vi "CameraSerialController_Experiment5555.vi"() -> (4 "图像时间戳":u32=16532020 format="%_32g")   [LabVIEW 2015]
uses:
  <vilib>/Instr/_visa.llb/VISA Configure Serial Port (Instr).vi
  MVCAMSDK.dll
  <vilib>/Analysis/NI_AALBase.lvlib
panel:
  out "光强图 4":dbl[](graph)
  out "variance 4":dbl caption="方差" format="%0.2f"
  out "光强图 3":dbl[](graph)
  out "variance 3":dbl caption="方差" format="%0.2f"
  out "连接的字符串":string
  out "转动信号曲线":cluster{"Locations":dbl[], "Amplitudes":dbl[]}[](graph)=[{"Locations"=array[750 elements], "Amplitudes"=array[749 elements]}, {"Locations"=[104.38621227921368, 258.3247060234782, 410.71523318402836, 562.6858730022967, 712.7065754646931], "Amplitudes"=[11153.698204083417, 10559.387052180104, 10974.865031894917, 10500.852817232146, 11059.763900010517]}, {"Locations"=[26.787398227992274, 182.39455189327623, 333.5517219531509, 488.1851999460032, 636.5270621135614], "Amplitudes"=[3284.809720018355, 2039.4564261182056, 3638.2587716464914, 3082.2730888167225, 4217.856016996603]}]
  in  "平移回退":T1=TRUE
  in  "转动回退":T1=TRUE
  in  "转动计数":u16
  in  "转动一次脉冲数":u16=20
  in  "转动前进":T1=TRUE
  in  "平移一次脉冲数":u16=20
  in  "平移计数":u16
  out "variance 2":dbl caption="方差" format="%0.2f"
  in  "flow control (0:none)":u16(ring) caption="流控制（0:无）" items=["无", "XON/XOFF", "RTS/CTS", "XON/XOFF & RTS/CTS", "DTR/DSR", "XON/XOFF & DTR/DSR"]
  in  "stop bits (10: 1 bit)":u16=10 caption="停止位（10: 1位）"
  in  "奇偶 (0:none)":enum16{"None", "Odd", "Even", "Mark", "Space"}(ring) caption="奇偶（0:无）"
  in  "数据比特(默认8)":u16(ring)=8 items=["5"=5, "6"=6, "7"=7, "8"=8]
  in  "波特率(默认9600)":u32=9600
  in  "端口":refnum<visa-resource-name>="COM1"
  in  "平移前进":T1=TRUE
  out "泰伯距离数值":dbl[](array[numeric])=[15.393849374426454, 15.239052716055017, 15.197063981826837, 15.002070246239633]
  out "Locations":dbl[](array[numeric])=[10.438621227921368, 25.832470602347822, 41.07152331840284, 56.268587300229676, 71.27065754646931] caption="上面图像曲线波峰位置"
  out "平移信号曲线":cluster{"Locations":dbl[], "Amplitudes":dbl[]}[](graph)=[{"Locations"=array[750 elements], "Amplitudes"=array[749 elements]}, {"Locations"=[104.38621227921368, 258.3247060234782, 410.71523318402836, 562.6858730022967, 712.7065754646931], "Amplitudes"=[11153.698204083417, 10559.387052180104, 10974.865031894917, 10500.852817232146, 11059.763900010517]}, {"Locations"=[26.787398227992274, 182.39455189327623, 333.5517219531509, 488.1851999460032, 636.5270621135614], "Amplitudes"=[3284.809720018355, 2039.4564261182056, 3638.2587716464914, 3082.2730888167225, 4217.856016996603]}]
  out "光强图 2":dbl[](graph)
  out "variance":dbl caption="方差" format="%0.2f"
  out "相机图像":T2(plugin-control)
  out "光强图":dbl[](graph)
  out "帧速":u32
  out "帧间耗时\n单位：（0.1ms）":u32
  in  "相机枚举":T3(ring)
  in  "自动曝光模式":bool=TRUE caption="软触发"
  in  "手动曝光模式":bool caption="软触发"
  in  "曝光时间，单位微秒":dbl=11000.0 format="%#_6f"
  in  "硬触发模式":bool caption="软触发"
  in  "软触发模式":bool caption="软触发"
  in  "连续模式":bool caption="软触发"
  in  "软触发一帧":bool caption="软触发"
  in  "读取自定义数据":bool
  out "从相机中读出的字符串(32字节)":string
  in  "写入自定义数据":bool
  in  "要写入相机的字符串(32字节)":string
  in  "拍照":bool
  in  "相机参数":bool=TRUE
  in  "Stop":bool
  in  "激活预览":bool=TRUE
  out "Image":T2(plugin-control)
  # "相机原生分辨率设置"
  # "写入自定义数据"
  # "触发设置"
  # "曝光设置"
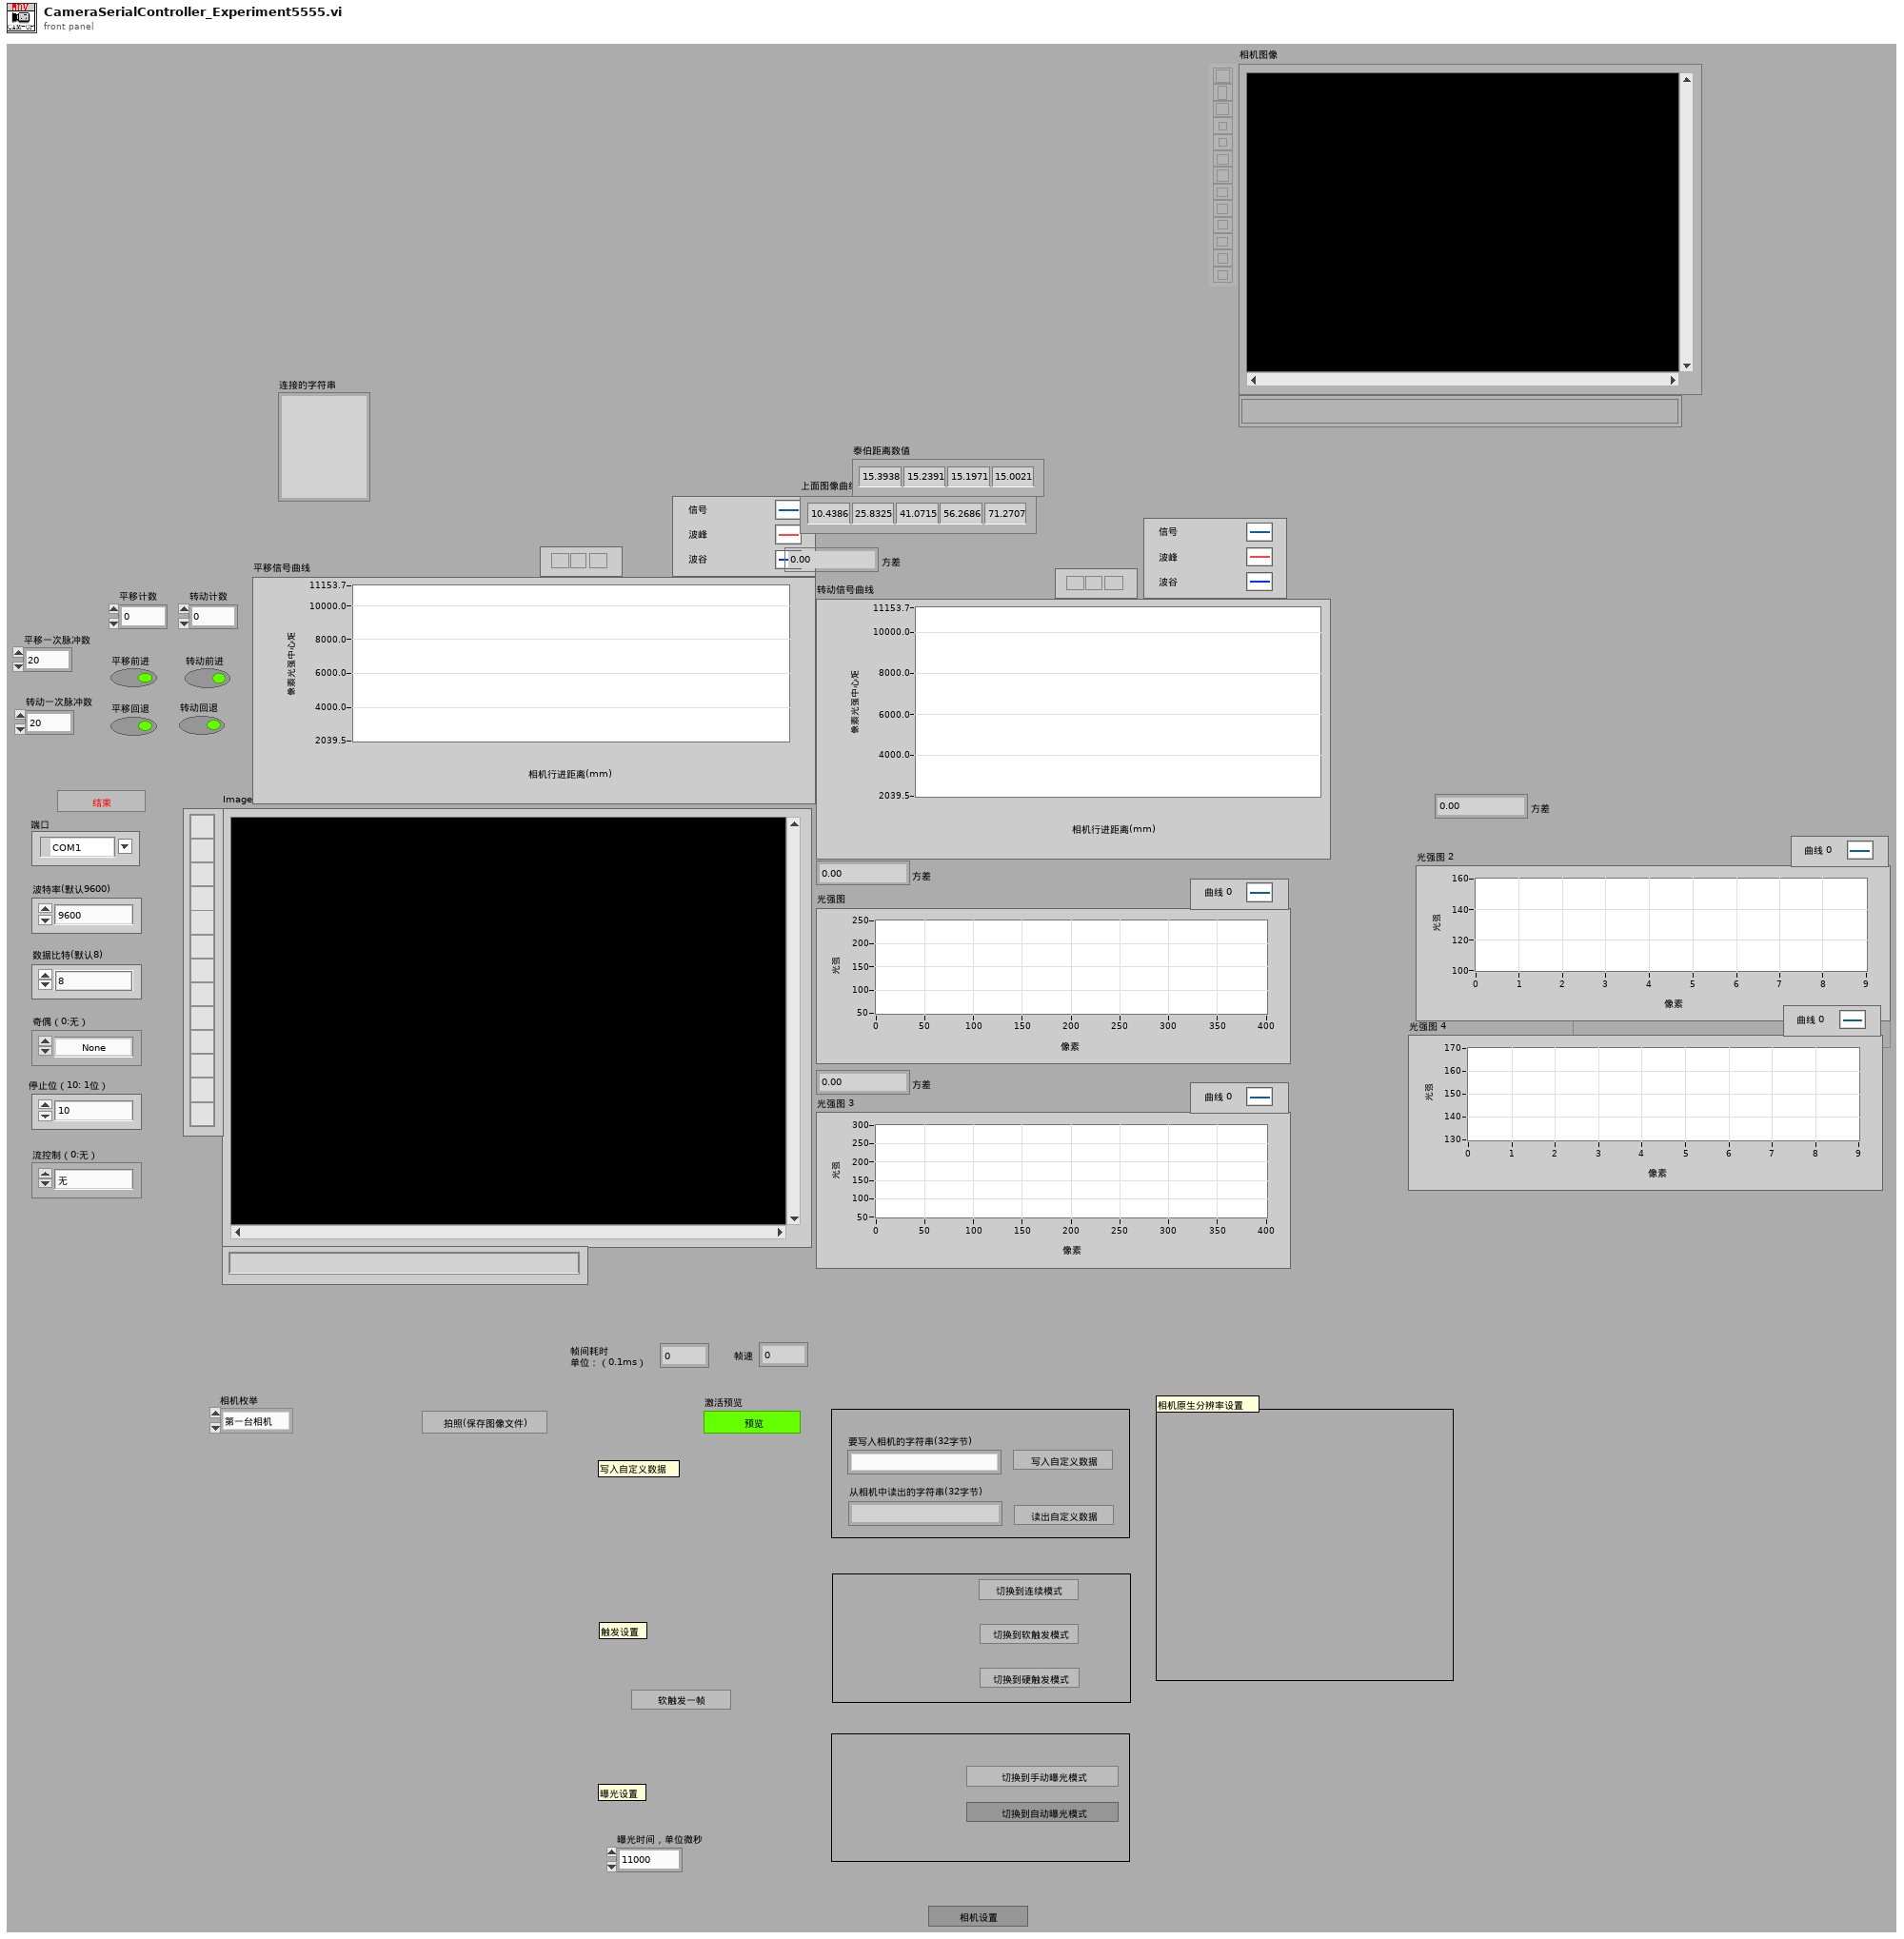
[diagram p1: front panel]
types:
  T1 = typedef "控件 1.ctl" = bool
  T2 = typedef "IMAQ Image.ctl" = refnum<image>
  T3 = enum16{"第一台相机", "第二台相机", "第三台相机", "第四台相机", "第五台相机"}
  T4 = typedef "Image Type" = u32
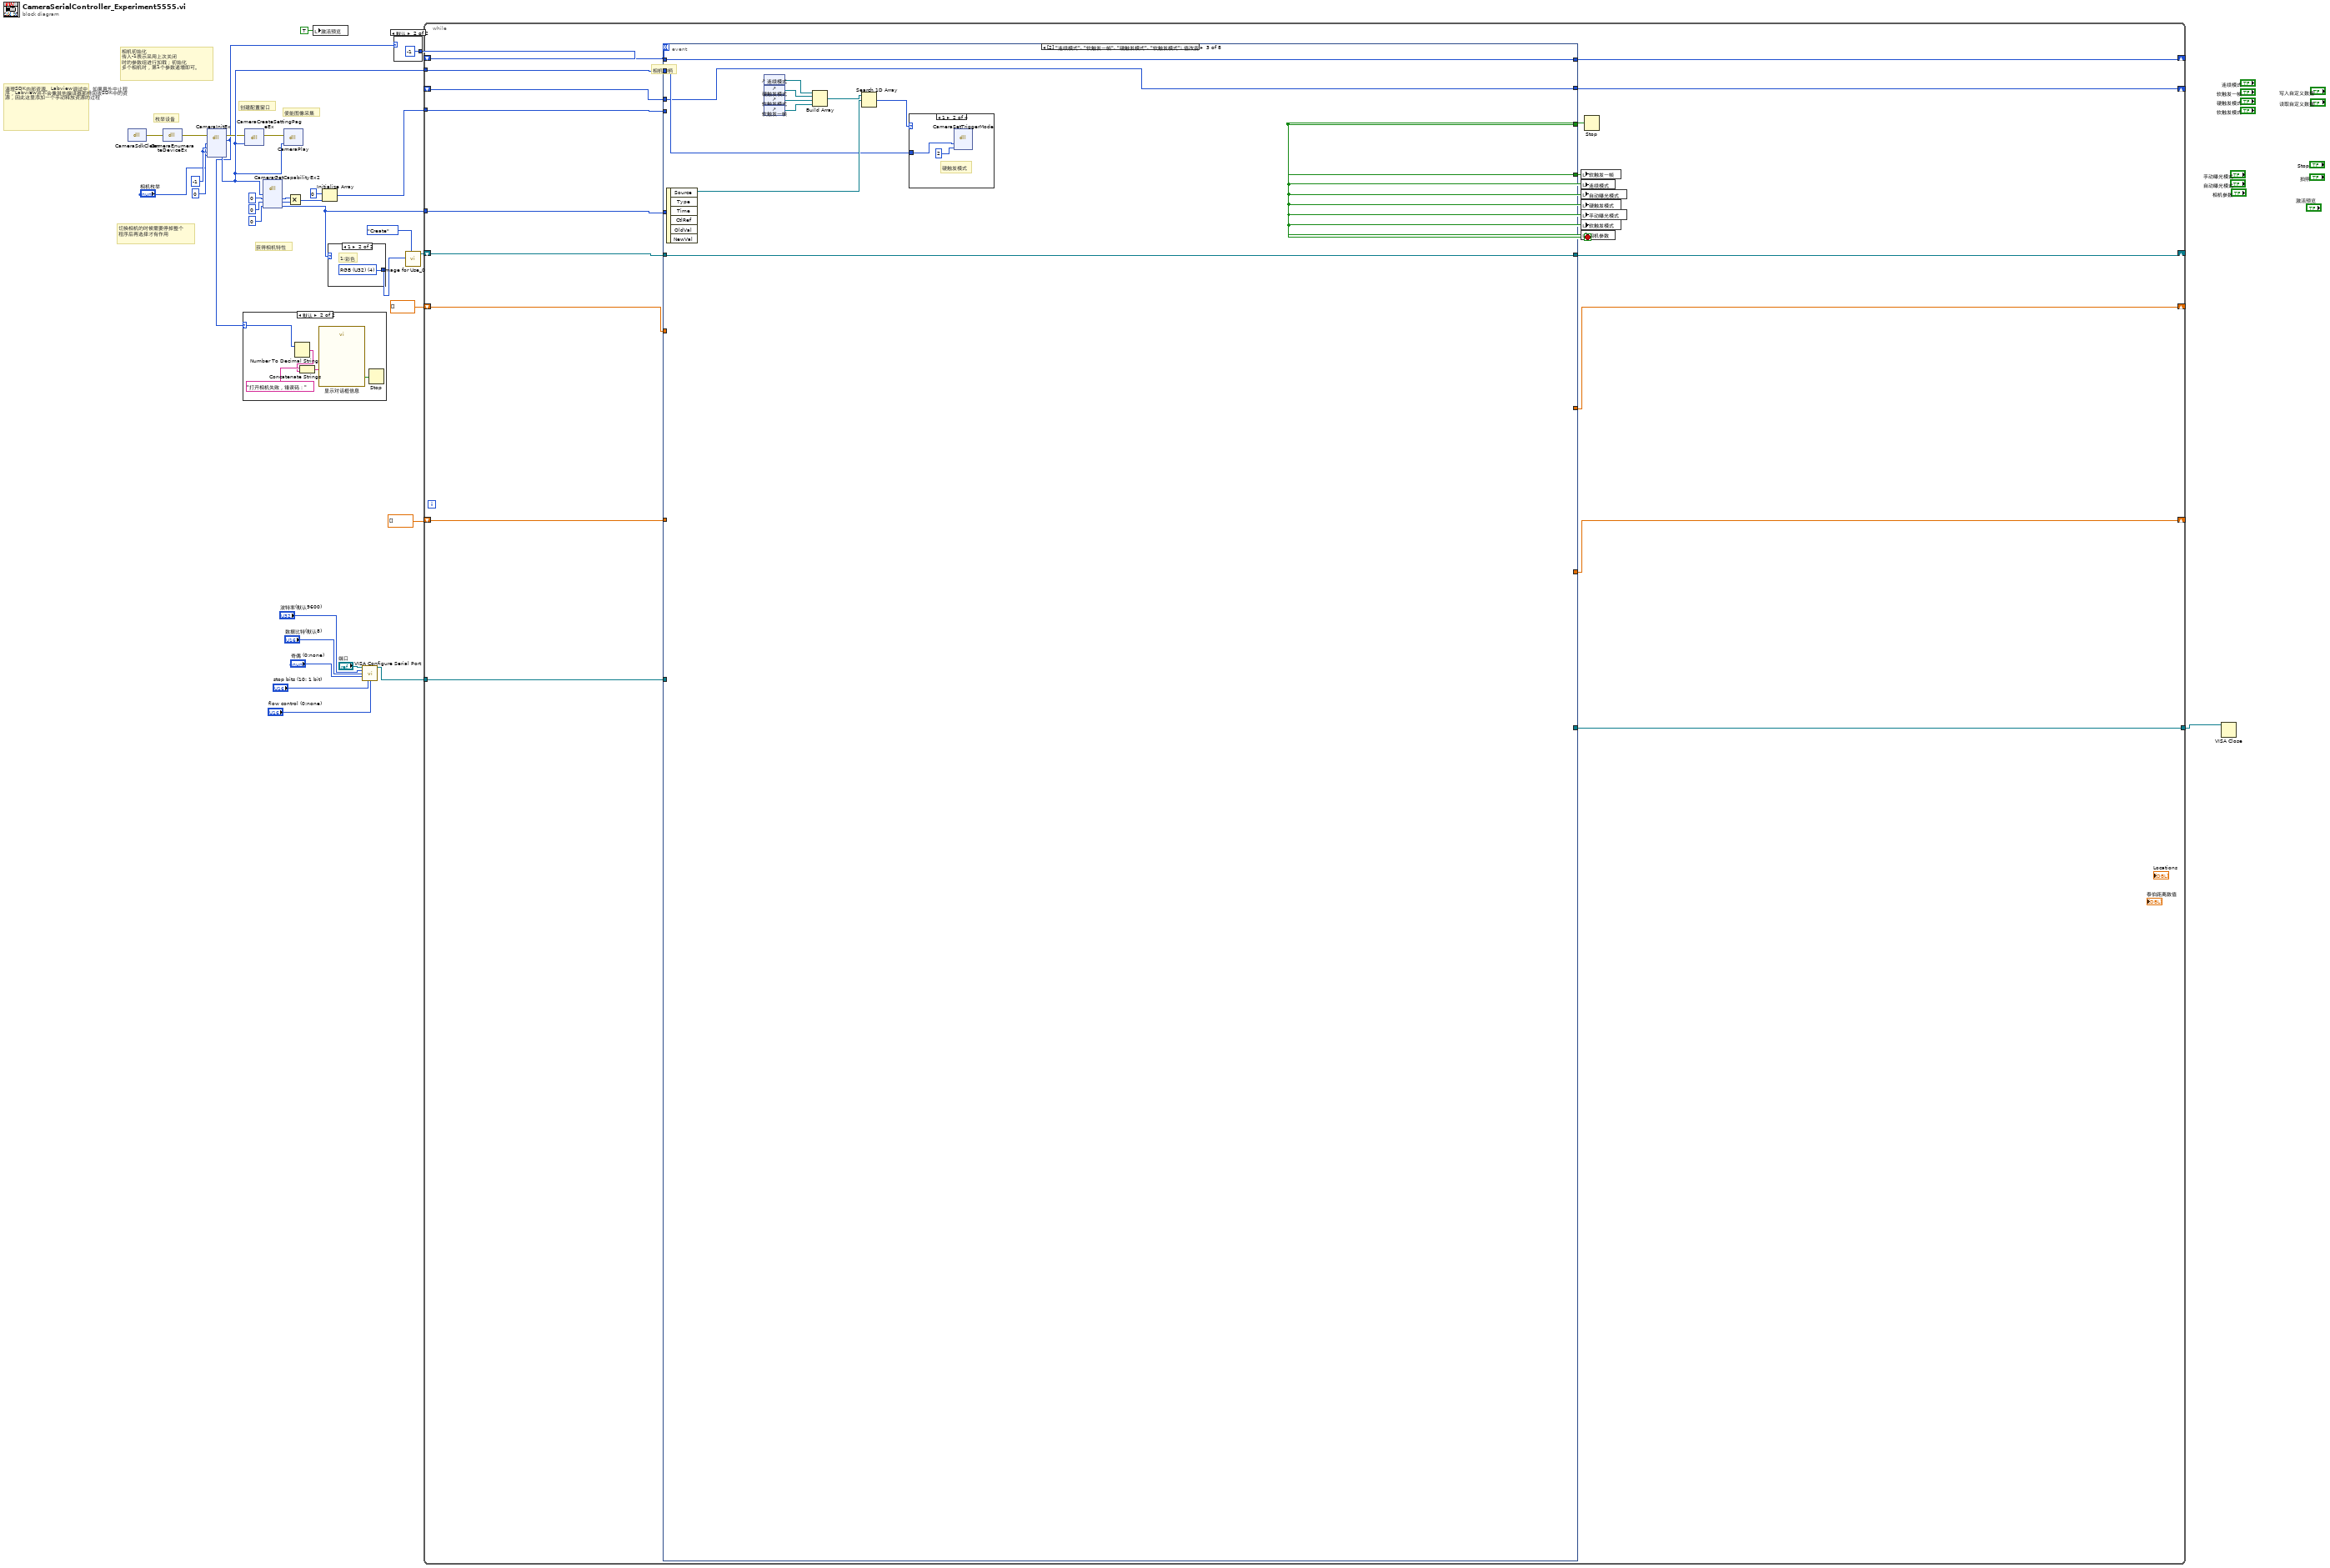
[diagram p0: block diagram]
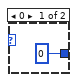
[diagram p2: hidden frame]
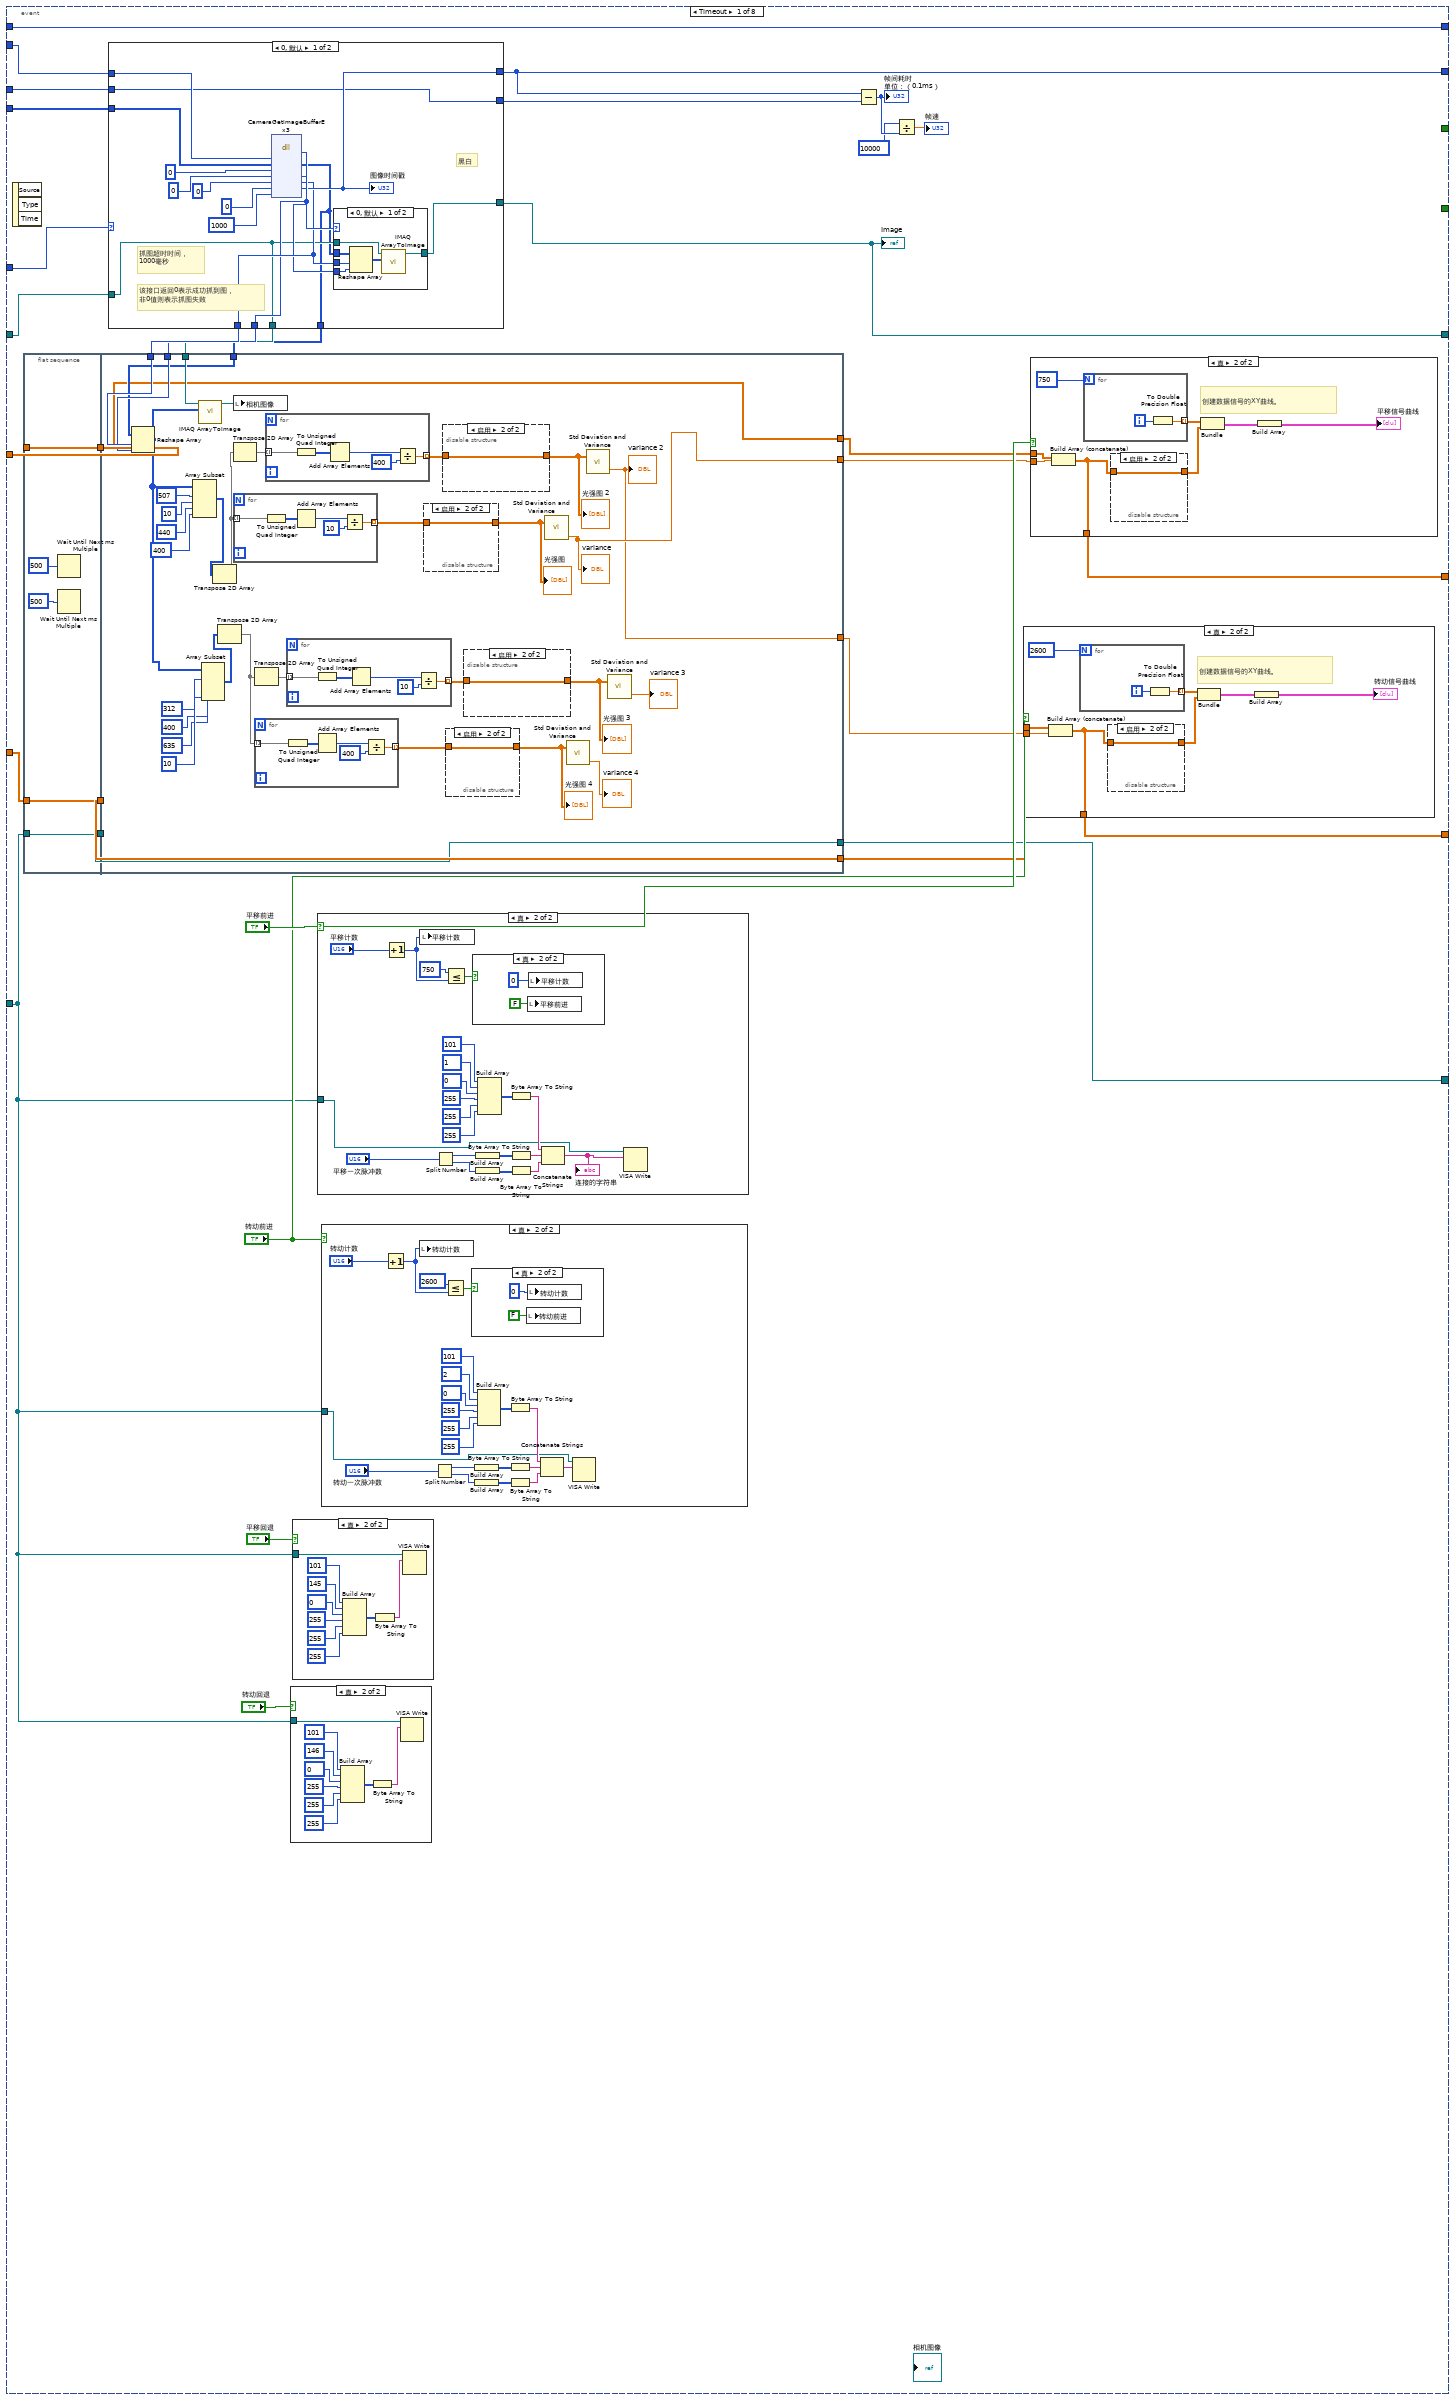
[diagram p4: hidden frame]
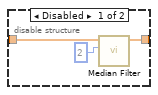
[diagram p5: hidden frame]
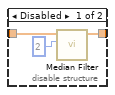
[diagram p6: hidden frame]
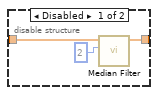
[diagram p7: hidden frame]
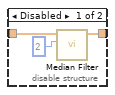
[diagram p8: hidden frame]
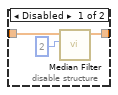
[diagram p10: hidden frame]
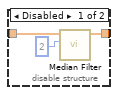
[diagram p12: hidden frame]
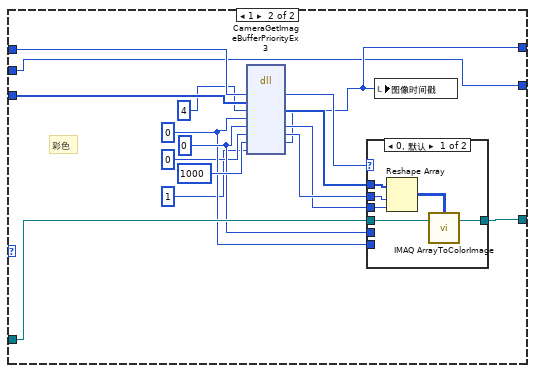
[diagram p20: hidden frame]
diagram:
  w30 = -1
  # "切换相机的时候需要停掉整个\n程序后再选择才有作用"
  # "清理SDK内部资源。Labview调试中，如果意外中止程序，Labview并不会像其他编译器那样回收SDK中的资源，因此这里添加一个手动释放资源的过程"
  # "使能图像采集"
  # "获得相机特性"
  # "创建配置窗口"
  # "相机初始化\n传入-1表示采用上次关闭\n时的参数组进行加载；初始化\n多个相机时，第1个参数递增即可。"
  # "枚举设备"
  n1 = dll-call lib="MVCAMSDK.dll" fn="CameraSdkClean"() -> (error out=w31:errorcluster)  [unwired: 4 in, 1 out]
  n2 = dll-call lib="MVCAMSDK.dll" fn="CameraEnumerateDeviceEx"(error in=w31) -> (error out=w28:errorcluster)  [unwired: 3 in, 1 out]
  n3 = dll-call lib="MVCAMSDK.dll" fn="CameraInitEx"(error in=w28, "相机索引值"="相机枚举", "参数加载方式"=w30, "要加载的参数组索引"=w30, "相机句柄"=0) -> (error out=w17:errorcluster, "返回类型"=w12:i32, "相机句柄"=w19:i32)  [unwired: 5 in, 1 out]
  n4 = case shown="默认" w12 {
    selector: w12 -> [_ w37]
    frame 0 {
    }
    frame Default {
      n5 = Number To Decimal String(number=w37) -> (decimal integer string=w34:string)  [unwired: 1 in]
      n6 = Concatenate Strings("打开相机失败，错误码：" ("字符串"), w34) -> (w36:string)
      n7 = call "显示对话框信息"("Message"=w36) -> ("结束"=w38:bool)  [unwired: 9 in, 1 out]
      n8 = Stop(stop? (T)=w38) -> ()
    }
  }
  n9 = dll-call lib="MVCAMSDK.dll" fn="CameraCreateSettingPageEx"(error in=w17, "相机句柄"=w19) -> (error out=w20:errorcluster)  [unwired: 4 in, 1 out]
  n10 = dll-call lib="MVCAMSDK.dll" fn="CameraGetCapabilityEx2"("相机句柄"=w19, "图像最大宽度"=0, "图像最大高度"=0, "是否是彩色相机(返回0:黑白;1:彩色)"=0) -> ("图像最大宽度"=w22:i32, "图像最大高度"=w21:i32, "是否是彩色相机(返回0:黑白;1:彩色)"=w16:i32)  [unwired: 5 in, 2 out]
  n11 = dll-call lib="MVCAMSDK.dll" fn="CameraPlay"(error in=w20, "相机句柄"=w19) -> ()  [unwired: 4 in, 2 out]
  n12 = Multiply(x=w22, y=w21) -> (x*y=w26:i32)
  n13 = local write "激活预览"(TRUE ("激活预览")) -> ()
  n14 = Initialize Array(0, w26) -> (w18:i32[])
  n15 = case shown="1" w16 {
    tunnel: [_ w39] -> w32
    frame 0, Default {
      # "0:黑白;"
    }
    frame 1 {
      w39 = T4 4 items=["Grayscale (U8)", "Grayscale (I16)", "Grayscale (SGL)", "Complex (CSG)", "RGB (U32)", "HSL (U32)", "RGB (U64)", "Grayscale (U16)"] ("Image Type")
      # "1:彩色"
    }
  }
  n16 = call-poly "VISA Configure Serial Port"("VISA resource name"="端口", "baud rate (9600)"="波特率(默认9600)", "data bits (8)"="数据比特(默认8)", "parity (0:none)"="奇偶 (0:none)", "stop bits (10: 1 bit)"="stop bits (10: 1 bit)", "flow control (0:none)"="flow control (0:none)") -> ("VISA resource name out"=w4:refnum<visa-resource-name>)  [unwired: 8 in, 1 out]
  n17 = case shown="默认" w12 {
    tunnel: [0 -1] -> w11
    frame 0 {
    }
    frame Default {
    }
  }
  n18 = call "Image for Use_0.vi"("Command"=enum16{"Create", "Use", "Copy in", "Dispose"}."Create", "Image Type"=w32) -> ("Image out"=w15:T2)  [unwired: 8 in, 1 out]
  n19 = while {
    tunnel: w19 -> [w55]
    tunnel: w18 -> [w57]
    tunnel: w16 -> [w58]
    shift-right: [w54] -> _
    shift-left: w11 -> [w53]
    shift-right: [w51] -> _
    shift-left: w15 -> [w56]
    shift-right: [w50] -> _
    shift-left: _ -> [w49]
    tunnel: w4 -> [w47]
    tunnel: [w46] -> w3
    shift-right: [w44] -> _
    shift-left: dbl[] [] -> [w45]
    shift-right: [w43] -> _
    shift-left: dbl[] [] -> [w42]
    stop <- w48 stop-if-true
    # "相机句柄"
    n20 = event shown="[2] \"连续模式\", \"软触发一帧\", \"硬触发模式\", \"软触发模式\": 值改变" {
      selector: _ -> [_ _ _ _ _ _ _ _]
      dyn-events: _ -> [_ _ _ _ _ _ _ _]
      timeout: w53 -> [_ _ _ _ _ _ _ _]
      tunnel: [_ _ _ _ _ _ _ TRUE] -> w48
      tunnel: w57 -> [w90 _ _ _ _ _ _ _]
      tunnel: w58 -> [w89 _ _ _ _ _ _ _]
      tunnel: w55 -> [w91 _ w315 w333 w348 _ w362 w382]
      tunnel: w56 -> [w88 w308 w314 w332 w347 w352 w361 w380]
      tunnel: [w87 w309 w316 w334 w349 w353 w363 w383] -> w54
      tunnel: w53 -> [w87 _ w316 w334 w349 w353 w363 w383]
      tunnel: [_ _ _ _ _ _ _ FALSE] -> w52
      tunnel: [w86 w308 w314 w332 w347 w352 w361 w380] -> w51
      tunnel: [w83 w307 w313 w331 w346 w351 w360 w379] -> w50
      tunnel: w49 -> [w85 w307 w313 w331 w346 w351 w360 w379]
      tunnel: w47 -> [w63 _ _ _ _ _ _ _]
      tunnel: [w62 _ _ _ _ _ _ _] -> w46
      tunnel: w45 -> [w69 _ _ _ _ _ _ _]
      tunnel: [w72 _ _ _ _ _ _ _] -> w44
      tunnel: [w71 _ _ _ _ _ _ _] -> w43
      tunnel: w42 -> [w65 _ _ _ _ _ _ _]
      event Timeout {
        n21 = event-data() -> ()  [unwired: 1 in, 3 out]
        n22 = flat-sequence {
          tunnel: w69 -> [w96]
          tunnel: [w96] -> w68
          tunnel: [w93] -> w66
          tunnel: w65 -> [w93]
          tunnel: [w92] -> w64
          tunnel: w63 -> [w92]
          tunnel: w79 -> [w130]
          tunnel: w78 -> [w129]
          tunnel: w77 -> [w128]
          tunnel: w76 -> [w127]
          tunnel: [w102] -> w60
          tunnel: [w117] -> w59
          tunnel: w68 -> [w117]
          tunnel: [w116] -> w67
          tunnel: w66 -> [w116]
          tunnel: [w115] -> w62
          tunnel: w64 -> [w115]
          tunnel: [w97] -> w61
          frame #0 {
            n23 = Wait Until Next ms Multiple(millisecond multiple=u32 500 ("毫秒倍数")) -> ()  [unwired: 1 out]
            n24 = Wait Until Next ms Multiple(millisecond multiple=u32 500 ("毫秒倍数")) -> ()  [unwired: 1 out]
          }
          frame #1 {
            n25 = Reshape Array(w127, w130, w129) -> (w104:u8[][])
            n26 = Array Subset(array=w104, index (row)=507 ("索引"), length (row)=10 ("长度"), index (col)=440 ("长度"), length (col)=400 ("索引")) -> (w99:u8[][])
            n27 = call "IMAQ ArrayToImage"("Image Pixels (U8)"=w104, "Image"=w128) -> ("Image Out"=w131:T2)  [unwired: 8 in, 1 out]
            n28 = Array Subset(array=w104, index (row)=312 ("索引"), length (row)=400 ("长度"), index (col)=635 ("长度"), length (col)=10 ("索引")) -> (w101:u8[][])
            n29 = Transpose 2D Array(2D array=w99) -> (transposed array=w98:u8[][])
            n30 = Transpose 2D Array(2D array=w101) -> (transposed array=w100:u8[][])
            n31 = local write "相机图像"(w131) -> ()
            n32 = Transpose 2D Array(2D array=w98) -> (transposed array=w124:u8[][])
            n33 = for {
              tunnel: w98 -> [w162] mode=indexing
              tunnel: [w160] -> w126 mode=indexing
              n34 = To Unsigned Quad Integer(1:w162) -> (0:w161:u64[])
              n35 = Add Array Elements(numeric array=w161) -> (sum=w163:u64)
              n36 = Divide(x=w163, y=u64 10) -> (x/y=w160:dbl)
            }
            n37 = Transpose 2D Array(2D array=w100) -> (transposed array=w108:u8[][])
            n38 = for {
              tunnel: w100 -> [w144] mode=indexing
              tunnel: [w142] -> w106 mode=indexing
              n39 = To Unsigned Quad Integer(1:w144) -> (0:w143:u64[])
              n40 = Add Array Elements(numeric array=w143) -> (sum=w145:u64)
              n41 = Divide(x=w145, y=u64 400) -> (x/y=w142:dbl)
            }
            n42 = for {
              tunnel: w124 -> [w153] mode=indexing
              tunnel: [w151] -> w125 mode=indexing
              n43 = To Unsigned Quad Integer(1:w153) -> (0:w152:u64[])
              n44 = Add Array Elements(numeric array=w152) -> (sum=w154:u64)
              n45 = Divide(x=w154, y=u64 400) -> (x/y=w151:dbl)
            }
            n46 = for {
              tunnel: w108 -> [w135] mode=indexing
              tunnel: [w133] -> w107 mode=indexing
              n47 = To Unsigned Quad Integer(1:w135) -> (0:w134:u64[])
              n48 = Add Array Elements(numeric array=w134) -> (sum=w136:u64)
              n49 = Divide(x=w136, y=u64 10) -> (x/y=w133:dbl)
            }
            n50 = disable-structure shown="启用" {
              disable-tunnel: w126 -> [w166 w167]
              disable-tunnel: [w164 w167] -> w123
              frame Disabled {
                n51 = call <vilib>:"Median Filter.vi"("left rank"=2, "X"=w166) -> ("Filtered X"=w164:dbl[])  [unwired: 8 in, 1 out]
              }
              frame Enabled {
              }
            }
            "光强图" <- w123
            n52 = disable-structure shown="启用" {
              disable-tunnel: w125 -> [w157 w158]
              disable-tunnel: [w155 w158] -> w122
              frame Disabled {
                n53 = call <vilib>:"Median Filter.vi"("left rank"=2, "X"=w157) -> ("Filtered X"=w155:dbl[])  [unwired: 8 in, 1 out]
              }
              frame Enabled {
              }
            }
            "光强图 2" <- w122
            n54 = disable-structure shown="启用" {
              disable-tunnel: w106 -> [w148 w149]
              disable-tunnel: [w146 w149] -> w109
              frame Disabled {
                n55 = call <vilib>:"Median Filter.vi"("left rank"=2, "X"=w148) -> ("Filtered X"=w146:dbl[])  [unwired: 8 in, 1 out]
              }
              frame Enabled {
              }
            }
            "光强图 4" <- w109
            n56 = disable-structure shown="启用" {
              disable-tunnel: w107 -> [w139 w140]
              disable-tunnel: [w137 w140] -> w110
              frame Disabled {
                n57 = call <vilib>:"Median Filter.vi"("left rank"=2, "X"=w139) -> ("Filtered X"=w137:dbl[])  [unwired: 8 in, 1 out]
              }
              frame Enabled {
              }
            }
            "光强图 3" <- w110
            n58 = call <vilib>:"Std Deviation and Variance.vi"("X"=w123) -> ("variance"=w102:dbl)  [unwired: 1 in, 2 out]
            "variance" <- w102
            n59 = call <vilib>:"Std Deviation and Variance.vi"("X"=w109) -> ("variance"=→"variance 4":dbl)  [unwired: 1 in, 2 out]
            n60 = call <vilib>:"Std Deviation and Variance.vi"("X"=w122) -> ("variance"=w97:dbl)  [unwired: 1 in, 2 out]
            "variance 2" <- w97
            n61 = call <vilib>:"Std Deviation and Variance.vi"("X"=w110) -> ("variance"=→"variance 3":dbl)  [unwired: 1 in, 2 out]
          }
        }
        n62 = case shown="0, 默认" w89 {
          tunnel: w90 -> [w276 w299]
          tunnel: w88 -> [w263 w298]
          tunnel: w91 -> [w268 w297]
          tunnel: [w269 w287] -> w86
          tunnel: [w267 w286] -> w83
          tunnel: w85 -> [w266 w285]
          tunnel: [w266 w285] -> w84
          tunnel: [w265 _] -> w79
          tunnel: [w264 _] -> w78
          tunnel: [w263 _] -> w77
          tunnel: [w262 _] -> w76
          frame 0, Default {
            # "黑白"
            # "该接口返回0表示成功抓到图，\n非0值则表示抓图失败"
            # "抓图超时时间，\n1000毫秒"
            n63 = dll-call lib="MVCAMSDK.dll" fn="CameraGetImageBufferEx3"("相机句柄"=w268, "图像数据缓冲区"=w276, "图像输出格式(0:8位灰度;1:24位彩色;2:32位彩色，3：BGR24彩色 4：BGRA32位彩色)"=0, "图像宽度"=0, "图像高度"=0, "时间戳(单位为100微秒)"=0, "抓图超时时间(毫秒)"=1000) -> ("返回类型"=w271:i32, "图像数据缓冲区"=w262:u8[], "图像宽度"=w264:i32, "图像高度"=w265:i32, "时间戳(单位为100微秒)"=w267:u32)  [unwired: 6 in, 2 out]
            "图像时间戳" <- w267
            n64 = case shown="0, 默认" w271 {
              tunnel: w262 -> [w282 _]
              tunnel: w263 -> [w279 w283]
              tunnel: w265 -> [w281 _]
              tunnel: w264 -> [w280 _]
              tunnel: [w277 w283] -> w269
              frame 0, Default {
                n65 = Reshape Array(w282, w281, w280) -> (w278:u8[][])
                n66 = call "IMAQ ArrayToImage"("Image Pixels (U8)"=w278, "Image"=w279) -> ("Image Out"=w277:T2)  [unwired: 8 in, 1 out]
              }
              frame -12 {
              }
            }
          }
          frame 1 {
            w289 = 0
            w290 = 0
            # "彩色"
            n67 = dll-call lib="MVCAMSDK.dll" fn="CameraGetImageBufferPriorityEx3"("相机句柄"=w297, "图像数据缓冲区"=w299, "图像输出格式(0:8位灰度;1:24位彩色;2:32位彩色)"=4, "图像宽度"=w289, "图像高度"=w290, "时间戳（单位为100微秒）"=0, "抓图超时时间(毫秒)"=1000, "取图优先级(0: 取最旧   1:取最新)"=1) -> ("返回类型"=w291:i32, "图像数据缓冲区"=w294:u32[], "图像宽度"=w292:i32, "图像高度"=w293:i32, "时间戳（单位为100微秒）"=w286:u32)  [unwired: 7 in, 2 out]
            n68 = case shown="0, 默认" w291 {
              tunnel: w294 -> [w304 _]
              tunnel: w298 -> [w303 w306]
              tunnel: w293 -> [w302 _]
              tunnel: w292 -> [w301 _]
              tunnel: w290 -> [_ _]
              tunnel: w289 -> [_ _]
              tunnel: [w300 w306] -> w287
              frame 0, Default {
                n69 = Reshape Array(w304, w302, w301) -> (w305:u32[][])
                n70 = call "IMAQ ArrayToColorImage"("Image Pixels (U32)"=w305, "Image"=w303) -> ("Image Out"=w300:T2)  [unwired: 3 in, 1 out]
              }
              frame -12 {
              }
            }
            n71 = local write "图像时间戳"(w286) -> ()
          }
        }
        "Image" <- w86
        n72 = case shown="真" "转动回退" {
          tunnel: w63 -> [_ w199]
          frame False {
          }
          frame True {
            n73 = Build Array(101, 146, 0, 255, 255, 255) -> (w200:i32[])
            n74 = Byte Array To String(unsigned byte array=w200) -> (string=w198:string)
            n75 = VISA Write(VISA resource name=w199, write buffer=w198) -> ()  [unwired: 1 in, 3 out]
          }
        }
        n76 = case shown="真" "平移回退" {
          tunnel: w63 -> [_ w208]
          frame False {
          }
          frame True {
            n77 = Build Array(101, 145, 0, 255, 255, 255) -> (w209:i32[])
            n78 = Byte Array To String(unsigned byte array=w209) -> (string=w207:string)
            n79 = VISA Write(VISA resource name=w208, write buffer=w207) -> ()  [unwired: 1 in, 3 out]
          }
        }
        n80 = case shown="真" "平移前进" {
          tunnel: w63 -> [_ w242]
          frame False {
          }
          frame True {
            n81 = Increment(x="平移计数") -> (x+1=w240:u16)
            n82 = local write "平移计数"(w240) -> ()
            n83 = Split Number(x="平移一次脉冲数") -> (hi(x)=w250:u8, lo(x)=w249:u8)
            n84 = Less Or Equal?(x=750, y=w240) -> (x <= y?=w252:bool)
            n85 = case shown="真" w252 {
              frame False {
              }
              frame True {
                n86 = local write "平移前进"(T1 FALSE ("平移前进")) -> ()
                n87 = local write "平移计数"(u16 0 ("平移计数 2")) -> ()
              }
            }
            n88 = Build Array(w250) -> (w248:u8[])
            n89 = Build Array(w249) -> (w247:u8[])
            n90 = Build Array(101, 1, 0, 255, 255, 255) -> (w246:i32[])
            n91 = Byte Array To String(unsigned byte array=w246) -> (string=w245:string)
            n92 = Byte Array To String(unsigned byte array=w248) -> (string=w244:string)
            n93 = Byte Array To String(unsigned byte array=w247) -> (string=w243:string)
            n94 = Concatenate Strings(w245, w244, w243) -> (w239:string)
            "连接的字符串" <- w239
            n95 = VISA Write(VISA resource name=w242, write buffer=w239) -> ()  [unwired: 1 in, 3 out]
          }
        }
        n96 = case shown="真" "转动前进" {
          tunnel: w63 -> [_ w220]
          frame False {
          }
          frame True {
            n97 = Increment(x="转动计数") -> (x+1=w218:u16)
            n98 = local write "转动计数"(w218) -> ()
            n99 = Split Number(x="转动一次脉冲数") -> (hi(x)=w228:u8, lo(x)=w227:u8)
            n100 = Less Or Equal?(x=2600, y=w218) -> (x <= y?=w230:bool)
            n101 = case shown="真" w230 {
              frame False {
              }
              frame True {
                n102 = local write "转动前进"(T1 FALSE ("平移前进")) -> ()
                n103 = local write "转动计数"(u16 0 ("平移计数")) -> ()
              }
            }
            n104 = Build Array(w228) -> (w226:u8[])
            n105 = Build Array(w227) -> (w225:u8[])
            n106 = Build Array(101, 2, 0, 255, 255, 255) -> (w224:i32[])
            n107 = Byte Array To String(unsigned byte array=w224) -> (string=w223:string)
            n108 = Byte Array To String(unsigned byte array=w226) -> (string=w222:string)
            n109 = Byte Array To String(unsigned byte array=w225) -> (string=w221:string)
            n110 = Concatenate Strings(w223, w222, w221) -> (w217:string)
            n111 = VISA Write(VISA resource name=w220, write buffer=w217) -> ()  [unwired: 1 in, 3 out]
          }
        }
        n112 = Subtract(x=w83, y=w84) -> (x-y=w82:u32)
        "帧间耗时\n单位：（0.1ms）" <- w82
        n113 = Divide(x=u32 10000 ("帧间耗时"), y=w82) -> (x/y=→"帧速":dbl)
        n114 = case shown="真" "转动前进" {
          tunnel: w61 -> [_ w171]
          tunnel: w67 -> [w168 w170]
          tunnel: [w168 w169] -> w71
          frame False {
          }
          frame True {
            # "创建数据信号的XY曲线。"
            n115 = Build Array (concatenate)(w170, w171) -> (w169:dbl[])
            n116 = for {
              N: i64 2600 ("数值") -> [_]
              tunnel: [w177] -> w173 mode=indexing
              i -> [w178]
              n117 = To Double Precision Float(number=w178) -> (double precision float=w177:dbl)
            }
            n118 = disable-structure shown="启用" {
              disable-tunnel: w169 -> [w180 w182]
              disable-tunnel: [w179 w182] -> w174
              frame Disabled {
                n119 = call <vilib>:"Median Filter.vi"("left rank"=2, "X"=w180) -> ("Filtered X"=w179:dbl[])  [unwired: 8 in, 1 out]
              }
              frame Enabled {
              }
            }
            n120 = Bundle(w173, w174) -> (w176:cluster{dbl[], dbl[]})  [unwired: 1 in]
            n121 = Build Array(w176) -> (→"转动信号曲线":cluster{dbl[], dbl[]}[])
          }
        }
        n122 = case shown="真" "平移前进" {
          tunnel: w59 -> [w183 w185]
          tunnel: w60 -> [_ w186]
          tunnel: [w183 w184] -> w72
          frame False {
          }
          frame True {
            # "创建数据信号的XY曲线。"
            n123 = Build Array (concatenate)(w185, w186) -> (w184:dbl[])
            n124 = for {
              N: i64 750 ("数值") -> [_]
              tunnel: [w192] -> w190 mode=indexing
              i -> [w193]
              n125 = To Double Precision Float(number=w193) -> (double precision float=w192:dbl)
            }
            n126 = disable-structure shown="启用" {
              disable-tunnel: w184 -> [w195 w197]
              disable-tunnel: [w194 w197] -> w189
              frame Disabled {
                n127 = call <vilib>:"Median Filter.vi"("left rank"=2, "X"=w195) -> ("Filtered X"=w194:dbl[])  [unwired: 8 in, 1 out]
              }
              frame Enabled {
              }
            }
            n128 = Bundle(w190, w189) -> (w187:cluster{dbl[], dbl[]})  [unwired: 1 in]
            n129 = Build Array(w187) -> (→"平移信号曲线":cluster{dbl[], dbl[]}[])
          }
        }
      }
      event "激活预览": Value Change {
        n130 = event-data() -> ("NewVal"=w310:bool)  [unwired: 1 in, 5 out]
        n131 = case shown="真" w310 {
          tunnel: [-1 0] -> w309
          frame False {
          }
          frame True {
          }
        }
      }
      event "连续模式", "软触发一帧", "硬触发模式", "软触发模式": Value Change {
        n132 = event-data() -> ("CtlRef"=w318:refnum<vi>)  [unwired: 1 in, 5 out]
        n133 = control-ref of="连续模式"() -> (w320:refnum<vi>)
        n134 = control-ref of="硬触发模式"() -> (w321:refnum<vi>)
        n135 = control-ref of="软触发模式"() -> (w322:refnum<vi>)
        n136 = control-ref of="软触发一帧"() -> (w323:refnum<vi>)
        n137 = Build Array ("创建数组")(w320, w321, w322, w323) -> (w319:refnum<vi>[])
        n138 = Search 1D Array(1D array=w319, element=w318) -> (index of element=w317:i32)  [unwired: 1 in]
        n139 = case shown="1" w317 {
          tunnel: w315 -> [w324 w326 w328 w330]
          frame 0, Default {
            # "连续模式"
            n140 = dll-call lib="MVCAMSDK.dll" fn="CameraSetTriggerMode"("相机句柄"=w324, "模式"=0) -> ()  [unwired: 6 in, 2 out]
          }
          frame 1 {
            # "硬触发模式"
            n141 = dll-call lib="MVCAMSDK.dll" fn="CameraSetTriggerMode"("相机句柄"=w326, "模式"=2) -> ()  [unwired: 6 in, 2 out]
          }
          frame 2 {
            # "软触发模式"
            n142 = dll-call lib="MVCAMSDK.dll" fn="CameraSetTriggerMode"("相机句柄"=w328, "模式"=1) -> ()  [unwired: 6 in, 2 out]
          }
          frame 3 {
            # "软触发一帧"
            n143 = dll-call lib="MVCAMSDK.dll" fn="CameraSoftTrigger"("相机句柄"=w330) -> ()  [unwired: 5 in, 2 out]
          }
        }
      }
      event "手动曝光模式", "自动曝光模式": Value Change {
        n144 = event-data() -> ("CtlRef"=w337:refnum<vi>)  [unwired: 1 in, 5 out]
        n145 = control-ref of="自动曝光模式"() -> (w335:refnum<vi>)
        n146 = control-ref of="手动曝光模式"() -> (w338:refnum<vi>)
        n147 = Build Array ("创建数组")(w338, w335) -> (w339:refnum<vi>[])
        n148 = Search 1D Array(1D array=w339, element=w337) -> (index of element=w336:i32)  [unwired: 1 in]
        n149 = case shown="0, 默认" w336 {
          tunnel: w333 -> [w340 w344]
          frame 0, Default {
            # "手动曝光模式"
            n150 = dll-call lib="MVCAMSDK.dll" fn="CameraSetAeState"("相机句柄"=w340, "曝光模式(0手动，1自动)"=0) -> (error out=w343:errorcluster)  [unwired: 6 in, 1 out]
            n151 = dll-call lib="MVCAMSDK.dll" fn="CameraSetExposureTime"(error in=w343, "相机句柄"=w340, "曝光时间，单位微秒"="曝光时间，单位微秒") -> ()  [unwired: 5 in, 2 out]
          }
          frame 1 {
            # "自动曝光模式"
            n152 = dll-call lib="MVCAMSDK.dll" fn="CameraSetAeState"("相机句柄"=w344, "曝光模式(0手动，1自动)"=1) -> ()  [unwired: 6 in, 2 out]
          }
        }
      }
      event "相机参数": Value Change {
        n153 = event-data() -> ()  [unwired: 1 in, 6 out]
        n154 = dll-call lib="MVCAMSDK.dll" fn="CameraShowSettingPage"("相机句柄"=w348, "状态"=TRUE) -> ()  [unwired: 6 in, 2 out]
      }
      event "拍照": Value Change {
        n155 = event-data() -> ()  [unwired: 1 in, 6 out]
        n156 = local read "Image"() -> (w354:T2)
        n157 = Format Date/Time String(time format string (%c)="%Y-%m-%d %H：%M：%S.bmp ") -> (date/time string=w358:string)  [unwired: 2 in]
        n158 = Concatenate Strings("c:\\", w358) -> (w355:string)
        n159 = String To Path(string=w355) -> (path=w357:path)
        n160 = call-poly "IMAQ Write File 2"("File Path"=w357, "Image"=w354) -> ()  [unwired: 8 in, 2 out]
      }
      event "写入自定义数据", "读取自定义数据": Value Change {
        n161 = event-data() -> ("CtlRef"=w365:refnum<vi>)  [unwired: 1 in, 5 out]
        n162 = control-ref of="读取自定义数据"() -> (w367:refnum<vi>)
        n163 = control-ref of="写入自定义数据"() -> (w366:refnum<vi>)
        n164 = Build Array ("创建数组")(w367, w366) -> (w368:refnum<vi>[])
        n165 = Search 1D Array(1D array=w368, element=w365) -> (index of element=w364:i32)  [unwired: 1 in]
        n166 = case shown="0, 默认" w364 {
          tunnel: w362 -> [w369 w376]
          frame 0, Default {
            n167 = Initialize Array(0, 32) -> (w373:i32[])
            n168 = dll-call lib="MVCAMSDK.dll" fn="CameraReadSN"("相机句柄"=w369, "序列号"=w373, "序列号级别，[0,1,2],0级为只读，1,2级可写"=1) -> ("序列号"=w371:u8[])  [unwired: 6 in, 2 out]
            n169 = Byte Array To String(unsigned byte array=w371) -> (string=→"从相机中读出的字符串(32字节)":string)
          }
          frame 1 {
            n170 = dll-call lib="MVCAMSDK.dll" fn="CameraWriteSN"("相机句柄"=w376, "序列号(固定为32个字节)"="要写入相机的字符串(32字节)", "序列号级别，[0,1,2]对应3级序列号，其中0级为只读，1,2级可写"=1) -> ()  [unwired: 7 in, 2 out]
          }
        }
      }
      event "Stop": Value Change {
        # "反初始化相机"
        n171 = event-data() -> ()  [unwired: 1 in, 6 out]
        n172 = dll-call lib="MVCAMSDK.dll" fn="CameraUnInit"("相机句柄"=w382) -> ()  [unwired: 5 in, 2 out]
      }
    }
    n173 = local write "软触发一帧"(w52) -> ()
    n174 = local write "连续模式"(w52) -> ()
    n175 = local write "自动曝光模式"(w52) -> ()
    n176 = local write "硬触发模式"(w52) -> ()
    n177 = local write "手动曝光模式"(w52) -> ()
    n178 = local write "软触发模式"(w52) -> ()
    n179 = local write "相机参数"(w52) -> ()
    n180 = Stop(stop? (T)=w48) -> ()
  }
  n181 = VISA Close(VISA resource name=w3) -> ()  [unwired: 1 in, 1 out]
